vi "Get Connection.vi"(11 "Processing in":refnum<class "Processing.lvclass">) -> (2 "Connection":refnum<class "HTTP TCP Client.lvclass">, 3 "Processing out":refnum<class "Processing.lvclass">)   [LabVIEW 2020, in "HTTP Server.lvlib" / "Processing.lvclass"]
uses:
  Processing.lvclass
  HTTP TCP Client/HTTP TCP Client.lvclass
  Processing.lvclass/Processing.ctl
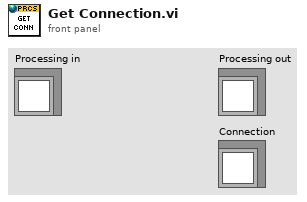
[diagram p1: front panel]
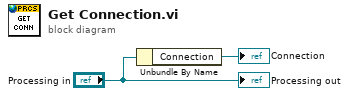
[diagram p0: block diagram]
diagram:
  n1 = Unbundle By Name("Processing in") -> ("Connection"=→"Connection":refnum<class "HTTP TCP Client.lvclass">)
  "Processing out" <- "Processing in"
